vi "EZ Digital.vi"(8 "error in (no error)":errorcluster, 9 "Byte/Word - Deprecated":bool, 10 "Scan List (empty)":string, 11 "VISA Resource Name":refnum<visa-resource-name>) -> (0 "error out":errorcluster, 2 "Output Array":u32[](array[numeric]), 3 "VISA Resource Name Out":refnum<visa-resource-name>)   [LabVIEW 2016, in "Agilent 34970.lvlib"]
doc: "This VI lets you take simple digital measurements.\n\n*Note* There was an bug in the old driver giving the option\nto read a word from the digital port. This is not possible\nwith the MEAS command. To read a word, according to\nthe documentation, put both digital input channels in the\nsame scan list. The readings will be taken simultaneously \nand given the same timestamp."
uses:
  Agilent 34970.lvlib
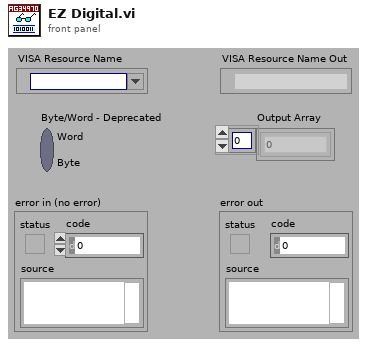
[diagram p1: front panel]
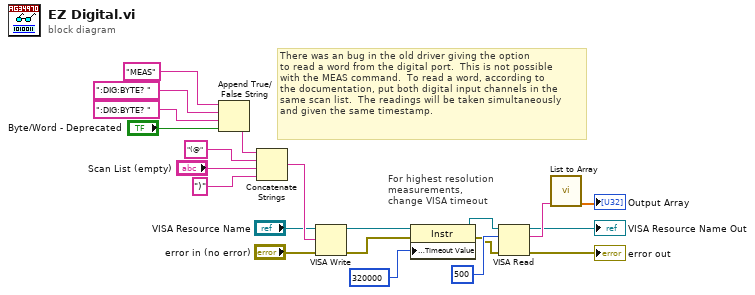
[diagram p0: block diagram]
diagram:
  # "For highest resolution\nmeasurements, \nchange VISA timeout"
  # "There was an bug in the old driver giving the option\nto read a word from the digital port.  This is not possible\nwith the MEAS command.  To read a word, according to\nthe documentation, put both digital input channels in the\nsame scan list.  The readings will be taken simultaneously \nand given the same timestamp."
  n1 = Append True/False String(1:"Byte/Word - Deprecated", 2:":DIG:BYTE? ", 3:":DIG:BYTE? ", 4:"MEAS") -> (0:w15:string)
  n2 = Concatenate Strings(w15, "(@", "Scan List (empty)", ")") -> (w14:string)
  n3 = VISA Write(VISA resource name="VISA Resource Name", write buffer=w14, error in (no error)="error in (no error)") -> (VISA resource name out=w4:refnum<visa-resource-name>, error out=w3:errorcluster)  [unwired: 1 out]
  n4 = property class="Instr"(reference=w4, error in=w3, "General Settings:Timeout Value"=u32 320000 ("Tmo Value")) -> (reference out=w1:refnum<visa-resource-name>, error out=w2:errorcluster)
  n5 = VISA Read(VISA resource name=w1, byte count=u32 500 ("byte count (0)"), error in (no error)=w2) -> (VISA resource name out=→"VISA Resource Name Out":refnum<visa-resource-name>, read buffer=w13:string, error out=→"error out":errorcluster)  [unwired: 1 out]
  n6 = call "List to Array.vi"("List (empty)"=w13) -> ("Output Number Array"=→"Output Array":dbl[])  [unwired: 9 in, 1 out]
